vi "Read Polling Ref.vi"(8 "error in (no error)":errorcluster, 11 "PRIME Detector in":refnum<class "PRIME Detector.lvclass">) -> (0 "error out":errorcluster, 2 "Polling Ref":refnum<k5>, 3 "PRIME Detector out":refnum<class "PRIME Detector.lvclass">)   [LabVIEW 2024, in "PRIME Detector.lvclass"]
uses:
  PRIME Detector.lvclass
  PRIME Detector.lvclass/PRIME Detector.ctl
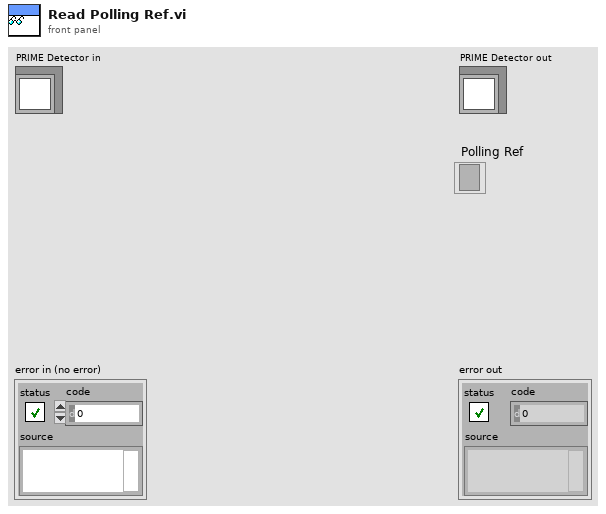
[diagram p1: front panel]
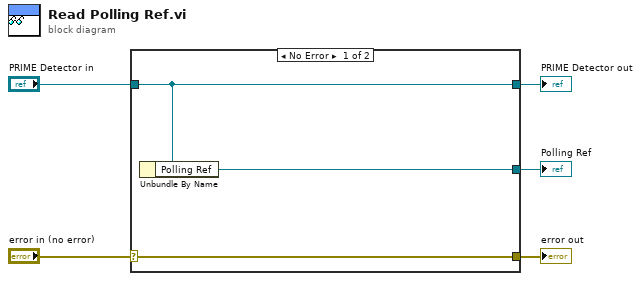
[diagram p0: block diagram]
diagram:
  n1 = case shown="No Error" "error in (no error)" {
    selector: "error in (no error)" -> [w8 w9]
    tunnel: [w8 w9] -> w4
    tunnel: [w7 w10] -> w2
    tunnel: "PRIME Detector in" -> [w7 w10]
    tunnel: [w6 _] -> w1
    frame No Error {
      n2 = Unbundle By Name(w7) -> ("Polling Ref"=w6:refnum<k5>)
    }
    frame Error {
    }
  }
  "error out" <- w4
  "PRIME Detector out" <- w2
  "Polling Ref" <- w1
